vi "1775E_User List.vi"(8 "Log?":bool, 11 "data":variant[][](array[variant])) -> ()   [LabVIEW 2020]
uses:
  <vilib>/Utility/miscctls.llb/LVRowAndColumnUnsignedTypeDef.ctl
panel:
  in  "Exit":bool
  in  "User list":i32(listbox)
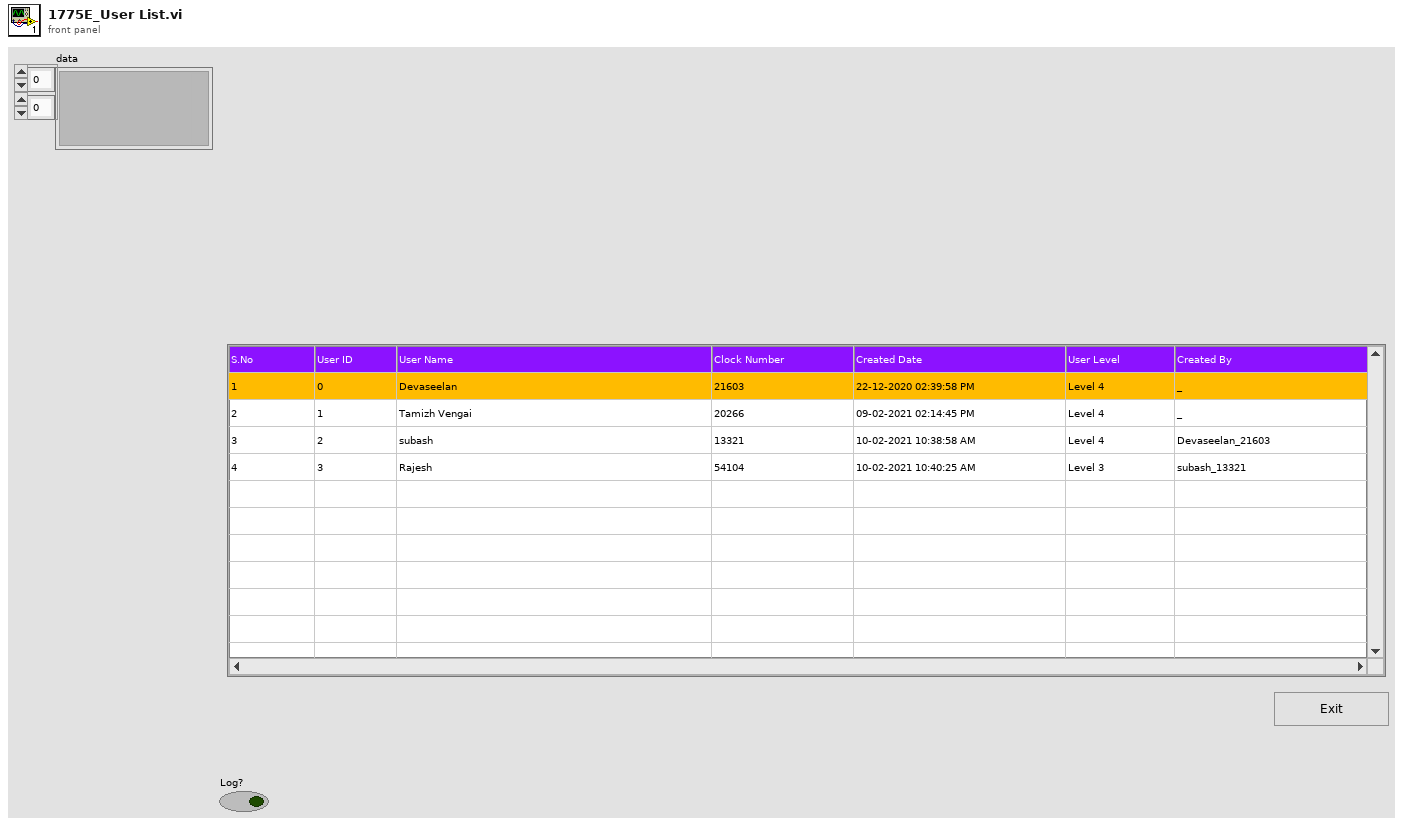
[diagram p1: front panel]
types:
  T1 = typedef "LVRowAndColumnUnsignedTypeDef.ctl" = cluster{"Row":u32, "Column":u32}
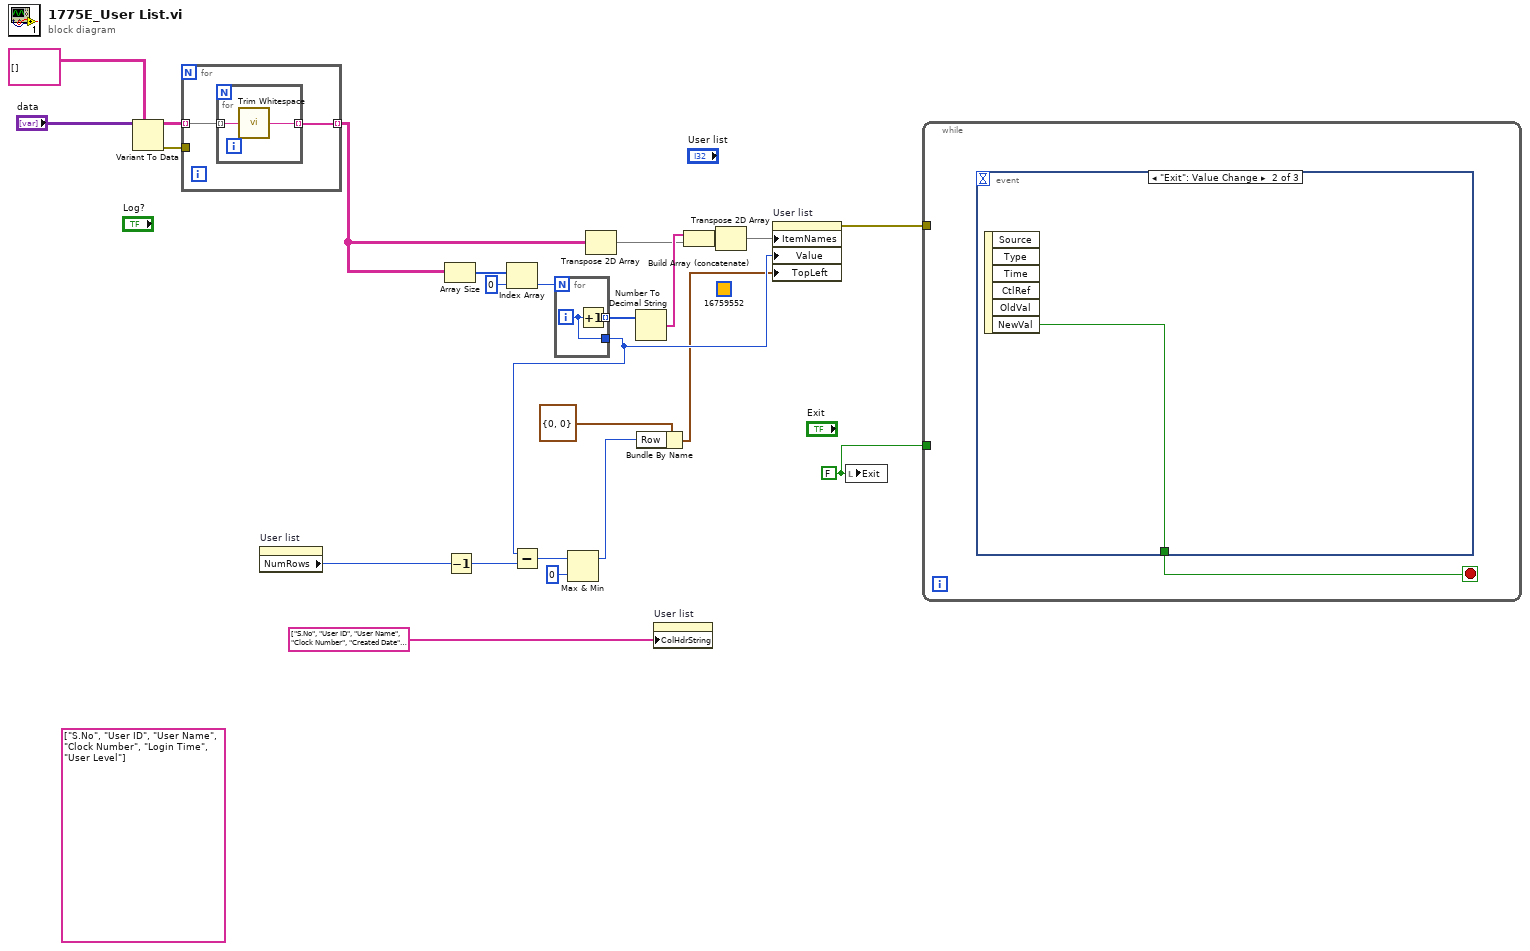
[diagram p0: block diagram]
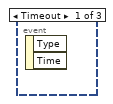
[diagram p2: hidden frame]
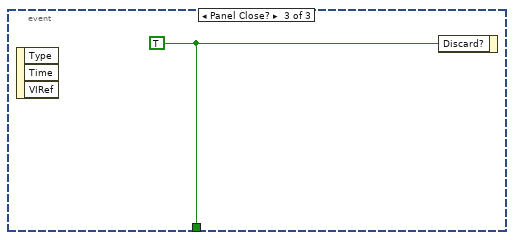
[diagram p3: hidden frame]
diagram:
  (unwired) u32 16759552 ("Selection Color")
  (unwired) string[] ["S.No", "User ID", "User Name", "Clock Number", "Login Time", "User Level"] ("Column Header Strings[]")
  w14 = FALSE ("Exit")
  n1 = Variant To Data(type=string[][] [] ("Array"), Variant="data") -> (data=w12:string[][], error out=w10:errorcluster)  [unwired: 1 in]
  n2 = for {
    tunnel: w12 -> [w26] mode=indexing
    tunnel: [w25] -> w11 mode=indexing
    tunnel: w10 -> [_]
    n3 = for {
      tunnel: w26 -> [w28] mode=indexing
      tunnel: [w27] -> w25 mode=indexing
      n4 = call <vilib>:"Trim Whitespace.vi"("string"=w28) -> ("trimmed string"=w27:string)  [unwired: 1 in]
    }
  }
  n5 = property on="User list" class="MCListbox (strict)"() -> ("NumRows"=w8:u32)  [unwired: 2 in, 2 out]
  n6 = Array Size(array=w11) -> (size(s)=w22:i32[])
  n7 = Decrement(x=w8) -> (x-1=w4:u32)
  n8 = Index Array(array=w22, index=0) -> (element=w20:i32)
  n9 = for {
    N: w20 -> [_]
    tunnel: [w30] -> w19 mode=indexing
    tunnel: [w29] -> w3
    i -> [w29]
    n10 = Increment(x=w29) -> (x+1=w30:i32)
  }
  n11 = Subtract(x=w3, y=w4) -> (x-y=w7:u32)
  n12 = Max & Min(x=w7, y=u32 0) -> (max(x,y)=w2:u32)  [unwired: 1 out]
  n13 = Transpose 2D Array(2D array=w11) -> (transposed array=w16:string[][])
  n14 = Number To Decimal String(number=w19) -> (decimal integer string=w17:string[])  [unwired: 1 in]
  n15 = Bundle By Name(cluster=T1 {"Row"=0, "Column"=0} ("Top Left Visible Cell"), "Row"=w2) -> (w1:T1)
  n16 = property on="User list" class="MCListbox (strict)"("ColHdrString"=string[] ["S.No", "User ID", "User Name", "Clock Number", "Created Date", "User Level", "Created By"] ("Column Header Strings[]")) -> ()  [unwired: 2 in, 2 out]
  n17 = Build Array (concatenate)(w17, w16) -> (w18:string[][])
  n18 = Transpose 2D Array(2D array=w18) -> (transposed array=w15:string[][])
  n19 = property on="User list" class="MCListbox (strict)"("ItemNames"=w15, "Value"=w3, "TopLeft"=w1) -> (error out=w13:errorcluster)  [unwired: 2 in, 1 out]
  n20 = local write "Exit"(w14) -> ()
  n21 = while {
    tunnel: w14 -> [_]
    tunnel: w13 -> [_]
    stop <- w31 stop-if-true
    n22 = event shown="[1] \"Exit\": Value Change" {
      selector: _ -> [_ _ _]
      dyn-events: _ -> [_ _ _]
      timeout: _ -> [_ _ _]
      tunnel: [_ w32 w33] -> w31
      event Timeout {
        n23 = event-data() -> ()  [unwired: 1 in, 2 out]
      }
      event "Exit": Value Change {
        n24 = event-data() -> ("NewVal"=w32:bool)  [unwired: 1 in, 5 out]
      }
      event Panel Close? {
        w33 = TRUE ("Discard?")
        n25 = event-data() -> ()  [unwired: 1 in, 3 out]
        n26 = event-data("Discard?"=w33) -> ()  [unwired: 1 in, 1 out]
      }
    }
  }
